vi "Signal Out High For Next Two Edges.vi"(4 "edge":bool, 5 "signal":bool) -> (1 "signal for distribution":bool)   [LabVIEW 2014, in "ni579x Synchronization v2 FPGA.lvlib"]
uses:
  <instrlib>/ni579x/Synchronization/v2/FPGA/ni579x Synchronization v2 FPGA.lvlib
  <instrlib>/_niInstr/Basic Elements/v1/FPGA/niInstr Basic Elements v1 FPGA.lvlib
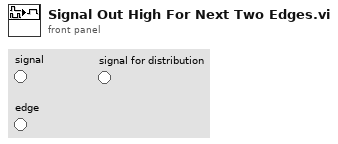
[diagram p1: front panel]
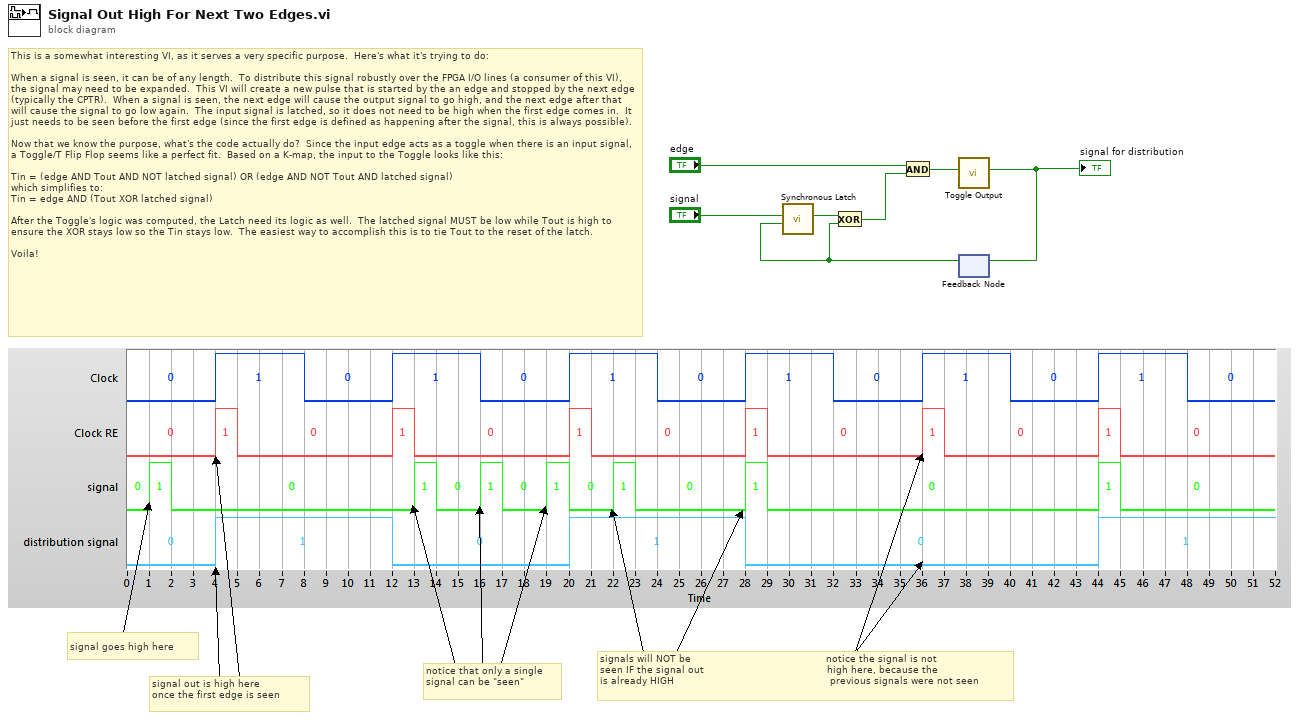
[diagram p0: block diagram]
diagram:
  # "signals will NOT be                                             notice the signal is not\nseen IF the signal out                                         high here, because the\nis already HIGH                                                    previous signals were not seen"
  # "notice that only a single\nsignal can be \"seen\""
  # "signal out is high here\nonce the first edge is seen"
  # "signal goes high here"
  # "This is a somewhat interesting VI, as it serves a very specific purpose.  Here's what it's trying to do:\n\nWhen a signal is seen, it can be of any length.  To distribute this signal robustly over the FPGA I/O lines (a consumer of this VI), the signal may need to be expanded.  This VI will create a new pulse that is started by the an edge and stopped by the next edge (typically the CPTR).  When a signal is seen, the next edge will cause the output signal to go high, and the next edge after that will cause the signal to go low again.  The input signal is latched, so it does not need to be high when the first edge comes in.  It just needs to be seen before the first edge (since the first edge is defined as happening after the signal, this is always possible).\n\nNow that we know the purpose, what's the code actually do?  Since the input edge acts as a toggle when there is an input signal, a Toggle/T Flip Flop seems like a perfect fit.  Based on a K-map, the input to the Toggle looks like this:\n\nTin = (edge AND Tout AND NOT latched signal) OR (edge AND NOT Tout AND latched signal)\nwhich simplifies to:\nTin = edge AND (Tout XOR latched signal)\n\nAfter the Toggle's logic was computed, the Latch need its logic as well.  The latched signal MUST be low while Tout is high to ensure the XOR stays low so the Tin stays low.  The easiest way to accomplish this is to tie Tout to the reset of the latch.\n\nVoila!"
  n1 = feedback #1() -> (w4:bool)  [unwired: 1 in]
  n2 = call <instrlib>:"Synchronous Latch.vi"("clear"=w4, "set"="signal") -> ("out"=w5:bool)  [unwired: 9 in]
  n3 = Exclusive Or(1:w4, 2:w5) -> (0:w7:bool)
  n4 = And(x="edge", y=w7) -> (x .and. y?=w2:bool)
  n5 = call <instrlib>:"Toggle Output.vi"("toggle"=w2) -> ("output"=w1:bool)  [unwired: 10 in]
  "signal for distribution" <- w1
  n6 = feedback-in #1(w1) -> ()
